vi "CopyAllDataByReference.vi"(8 "error in (no error)":errorcluster) -> (0 "error out":errorcluster, 2 "data0":u16[](array[numeric]))   [LabVIEW 2015, in "ESLSCDLL.lvlib"]
uses:
  ESLSCDLL.lvlib
  Globals.vi
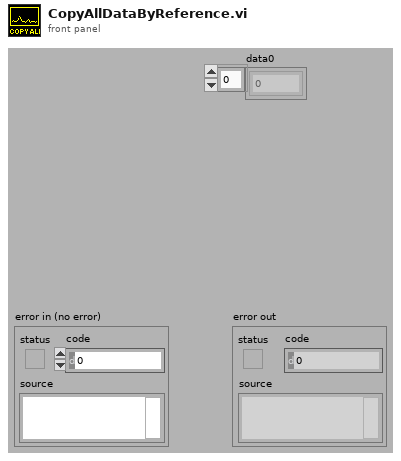
[diagram p1: front panel]
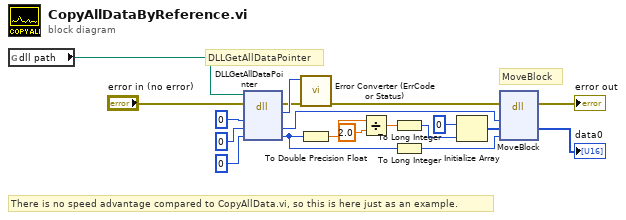
[diagram p0: block diagram]
diagram:
  # "There is no speed advantage compared to CopyAllData.vi, so this is here just as an example."
  # "DLLGetAllDataPointer"
  # "MoveBlock"
  n1 = global read "Globals.vi" "dll path"() -> (w1:path)
  n2 = dll-call lib="C:/ENTW/PCIE/LV64/board.vis/ESLSCDLL.dll" fn="DLLGetAllDataPointer" ("lwlscdll.dll:DLLReadLongS0")(path in=w1, error in="error in (no error)", "drvno"=u32 0, "pdest"=i64 0, "bytes_to_end_of_buffer"=u64 0) -> (error out=w3:errorcluster, "Rückgabetyp"=w4:i32, "pdest"=w14:i64, "bytes_to_end_of_buffer"=w6:u64)  [unwired: 2 in, 1 out]
  n3 = call "Error Converter (ErrCode or Status).vi"("error in (no error)"=w3, "error code"=w4) -> ("error out"=w2:errorcluster)  [unwired: 9 in]
  n4 = To Double Precision Float(number=w6) -> (double precision float=w9:dbl)
  n5 = Divide(x=w9, y=2.0) -> (x/y=w7:dbl)
  n6 = To Long Integer(number=w7) -> (32bit integer=w18:i32)
  n7 = To Long Integer(number=w6) -> (32bit integer=w11:i32)
  n8 = Initialize Array(u16 0, w18) -> (w13:u16[])
  n9 = dll-call lib="LabVIEW" fn="MoveBlock" ("lwlscdll.dll:DLLReadLongS0")(error in=w2, "Address (Pointer)"=w14, "Destination"=w13, "Size"=w11) -> (error out=→"error out":errorcluster, "Destination"=→"data0":u16[])  [unwired: 5 in, 1 out]
